vi "mainControlSerial.vi"(8 "error in (no error)":errorcluster, 10 "Queue In":T1) -> (0 "error out":errorcluster)   [LabVIEW 2014, in "LibraryGcode.lvlib"]
uses:
  LibraryGcode.lvlib
  control/Queue/QueueCMDandPOS.ctl
  control/Queue/TypeDataPOS.ctl
  control/stateCmdUpdatePara.ctl
  <vilib>/Platform/TimedLoop/XDataNode/timing_clust.ctl
  <vilib>/Platform/TimedLoop/XDataNode/nitl_modes.ctl
  <vilib>/Platform/TimedLoop/XDataNode/wakeup.ctl
  ClassUART/GiaoTiepUART.lvclass
  control/TypeFirmwareControl.ctl
  ClassUART/StateMachine_UART.ctl
  variableGlobal/StartAutoandGcode.vi
  <vilib>/Platform/TimedLoop/XDataNode/XDataNode.xnode
  <vilib>/Platform/TimedLoop/XDataNode/XDNodeRunTimeDep.lvlib
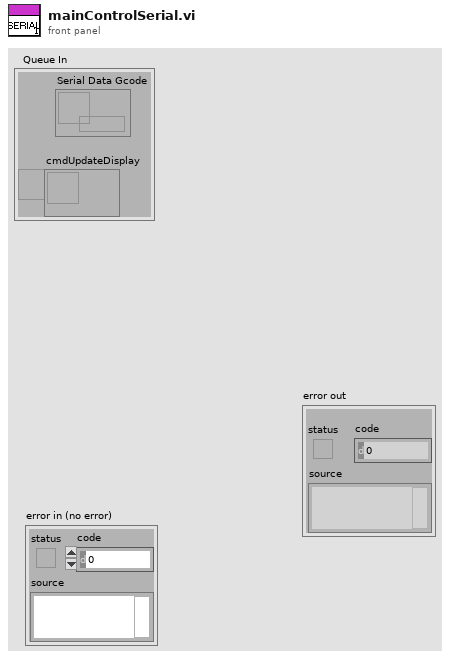
[diagram p1: front panel]
types:
  T1 = typedef "LibraryGcode.lvlib/QueueCMDandPOS.ctl" = cluster{"Serial Data Gcode":refnum<queue>, "cmdUpdateDisplay":refnum<queue>}
  T2 = typedef "LibraryGcode.lvlib/TypeFirmwareControl.ctl" = enum16{"ScaraMarlin", "CncMarlin", "Mk4Due"}
  T3 = typedef "XDNodeRunTimeDep.lvlib/timing_clust.ctl" = cluster{"Expected End [f-1]":u64, "Actual End [f-1]":u64, "Finished Late? [f-1]":bool, "Expected End [i-1]":u64, "Actual End [i-1]":u64, "Finished Late? [i-1]":bool, "Expected Start [i]":u64, "Actual Start [i]":u64, "Expected Start [f]":u64, "Actual Start [f]":u64, "Source Name":string, "Structure Name":string, "Period":i64, "Deadline":i64, "Offset":i64, "Start":i64, "Priority":i32, "Timeout":i32, "Mode":T4, "Wakeup Reason":T5, "Error":errorcluster, "Source Type":string, "Secondary Source Type":string, "Global End Time":u64, "Global Start Time":u64, "Frame Duration":u64, "Iteration Duration":u64, "Assigned CPU":i32, "I/O Scan Engine Mode":u32}
  T4 = typedef "XDNodeRunTimeDep.lvlib/nitl_modes.ctl" = enum32{"No Change", "Process missed periods, maintain original phase", "Discard missed periods, maintain original phase", "Process missed periods, ignore original phase", "Discard missed periods, ignore original phase"}
  T5 = typedef "XDNodeRunTimeDep.lvlib/wakeup.ctl" = enum32{"Normal", "Aborted", "Asynchronous wakeup", "Timing source error", "Timed loop error", "Timeout"}
  T6 = typedef "LibraryGcode.lvlib/GiaoTiepUART.lvclass/StateMachine_UART.ctl" = enum16{"INIT", "WRITE", "READ", "CHECKDATA", "IDLE", "STOP"}
  T7 = typedef "LibraryGcode.lvlib/stateBoardFirmware.ctl" = enum16{"Running", "Waiting", "Pos", "IDLE"}
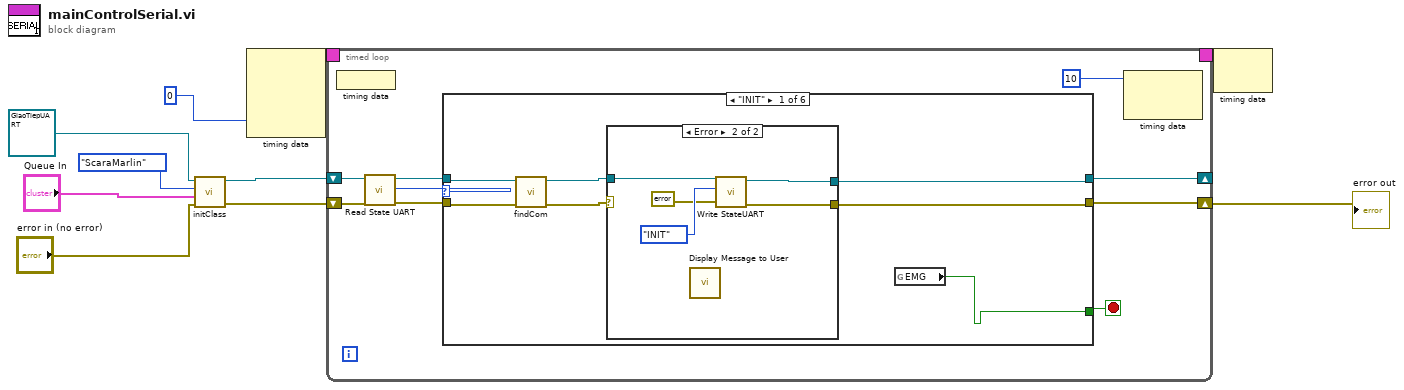
[diagram p0: block diagram]
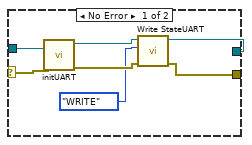
[diagram p2: hidden frame]
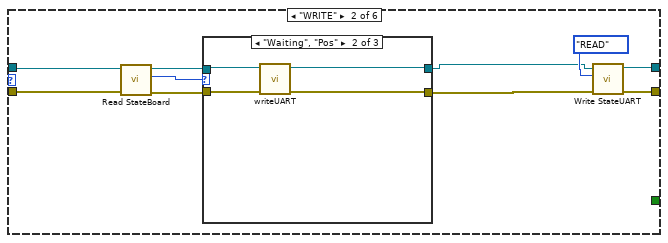
[diagram p3: hidden frame]
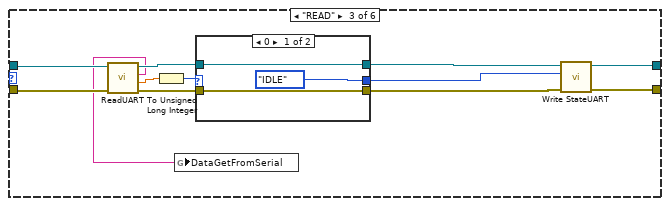
[diagram p6: hidden frame]
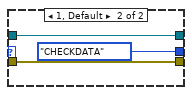
[diagram p7: hidden frame]
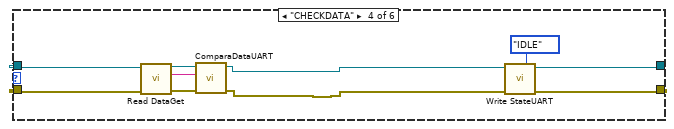
[diagram p8: hidden frame]
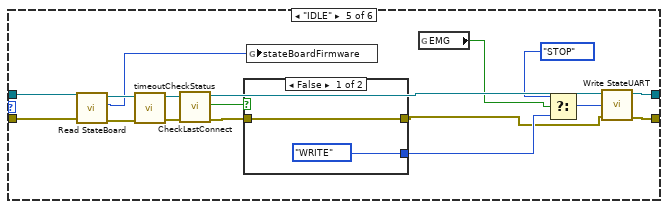
[diagram p9: hidden frame]
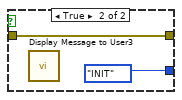
[diagram p10: hidden frame]
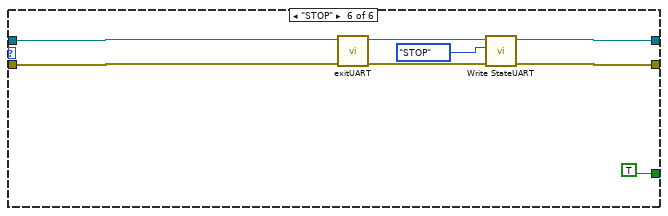
[diagram p11: hidden frame]
diagram:
  n1 = call-dynamic "initClass.vi"("error un"="error in (no error)", "Queue In"="Queue In", "TypeFirmware"=TypeFirmwareControl."ScaraMarlin", "GiaoTiepUART in"=refnum<class "GiaoTiepUART.lvclass"> refnum) -> ("error out"=w5:errorcluster, "GiaoTiepUART out"=w6:refnum<class "GiaoTiepUART.lvclass">)  [unwired: 6 in]
  n2 = node-c288(0 ("Processor")) -> (w10:T3)  [unwired: 3 in]
  n3 = timed-loop {
    timing: w10 -> [_]
    timing-out: [_] -> w9
    shift-right: [w18] -> _
    shift-left: w6 -> [w15]
    shift-right: [w17] -> w7
    shift-left: w5 -> [w16]
    stop <- w11 stop-if-true
    n4 = node-c288() -> ()  [unwired: 1 in]
    n5 = call-dynamic "Read State UART.vi"("error in (no error)"=w16, "GiaoTiepUART in"=w15) -> ("error out"=w13:errorcluster, "STATEUART"=w12:T6, "GiaoTiepUART out"=w14:refnum<class "GiaoTiepUART.lvclass">)  [unwired: 7 in]
    n6 = case shown="\"INIT\"" w12 {
      tunnel: [w20 _ _ _ _ TRUE] -> w11
      tunnel: [w26 w47 w66 w84 w97 w113] -> w18
      tunnel: w14 -> [w23 w42 w68 w81 w91 w106]
      tunnel: w13 -> [w22 w41 w67 w80 w89 w108]
      tunnel: [w21 w46 w65 w83 w96 w109] -> w17
      frame "INIT" {
        n7 = call-dynamic "findCom.vi"("error in (no error)"=w22, "GiaoTiep in"=w23) -> ("error out"=w25:errorcluster, "GiaoTiep out"=w24:refnum<class "GiaoTiepUART.lvclass">)  [unwired: 8 in]
        n8 = case shown="Error" w25 {
          selector: w25 -> [w33 _]
          tunnel: [w30 w36] -> w26
          tunnel: w24 -> [w32 w38]
          tunnel: [w31 w35] -> w21
          frame No Error {
            n9 = call-dynamic "initUART.vi"("error in (no error)"=w33, "GiaoTiep in"=w32) -> ("error out"=w28:errorcluster, "GiaoTiep out"=w29:refnum<class "GiaoTiepUART.lvclass">)  [unwired: 8 in]
            n10 = call-dynamic "Write StateUART.vi"("error in (no error)"=w28, "STATEUART"=StateMachine_UART."WRITE", "GiaoTiepUART in"=w29) -> ("error out"=w31:errorcluster, "GiaoTiepUART out"=w30:refnum<class "GiaoTiepUART.lvclass">)  [unwired: 7 in]
          }
          frame Error {
            n11 = call "Display Message to User"() -> ()  [unwired: 10 in, 2 out]
            n12 = call-dynamic "Write StateUART.vi"("error in (no error)"=errorcluster {"status"=FALSE, "code"=30011991, "source"="NoConnect "}, "STATEUART"=StateMachine_UART."INIT", "GiaoTiepUART in"=w38) -> ("error out"=w35:errorcluster, "GiaoTiepUART out"=w36:refnum<class "GiaoTiepUART.lvclass">)  [unwired: 7 in]
          }
        }
        n13 = global read "StartAutoandGcode.vi" "EMG"() -> (w20:bool)
      }
      frame "WRITE" {
        n14 = call-dynamic "Read StateBoard.vi"("error in (no error)"=w41, "XuLyStringUART in"=w42) -> ("error out"=w43:errorcluster, "StatePos"=w40:T7, "XuLyStringUART out"=w44:refnum<class "GiaoTiepUART.lvclass">)  [unwired: 7 in]
        n15 = case shown="\"Waiting\", \"Pos\"" w40 {
          tunnel: w44 -> [w50 w54 w56]
          tunnel: [w50 w52 w56] -> w39
          tunnel: w43 -> [w49 w53 w55]
          tunnel: [w49 w51 w55] -> w48
          frame "Running", Default {
          }
          frame "Waiting", "Pos" {
            n16 = call-dynamic "writeUART.vi"("error in (no error)"=w53, "GiaoTiep in"=w54) -> ("error out"=w51:errorcluster, "GiaoTiep out"=w52:refnum<class "GiaoTiepUART.lvclass">)  [unwired: 7 in, 1 out]
          }
          frame "IDLE" {
          }
        }
        n17 = call-dynamic "Write StateUART.vi"("error in (no error)"=w48, "STATEUART"=StateMachine_UART."READ", "GiaoTiepUART in"=w39) -> ("error out"=w46:errorcluster, "GiaoTiepUART out"=w47:refnum<class "GiaoTiepUART.lvclass">)  [unwired: 7 in]
      }
      frame "READ" {
        n18 = call-dynamic "ReadUART.vi"("error in (no error)"=w67, "GiaoTiep in"=w68) -> ("error out"=w62:errorcluster, "milisecondGetData"=w59:dbl, "read buffer"=w57:string, "GiaoTiep out"=w61:refnum<class "GiaoTiepUART.lvclass">)  [unwired: 6 in]
        n19 = To Unsigned Long Integer(number=w59) -> (unsigned 32bit integer=w58:u32)
        n20 = global write "StartAutoandGcode.vi" "DataGetFromSerial"(w57) -> ()
        n21 = case shown="0" w58 {
          tunnel: [StateMachine_UART."IDLE" StateMachine_UART."CHECKDATA"] -> w64
          tunnel: [w70 w73] -> w63
          tunnel: w62 -> [w70 w73]
          tunnel: [w69 w72] -> w60
          tunnel: w61 -> [w69 w72]
          frame 0 {
          }
          frame 1, Default {
          }
        }
        n22 = call-dynamic "Write StateUART.vi"("error in (no error)"=w63, "STATEUART"=w64, "GiaoTiepUART in"=w60) -> ("error out"=w65:errorcluster, "GiaoTiepUART out"=w66:refnum<class "GiaoTiepUART.lvclass">)  [unwired: 7 in]
      }
      frame "CHECKDATA" {
        n23 = call-dynamic "Read DataGet.vi"("error in (no error)"=w80, "GiaoTiepUART in"=w81) -> ("error out"=w78:errorcluster, "DataGet"=w77:string, "GiaoTiepUART out"=w79:refnum<class "GiaoTiepUART.lvclass">)  [unwired: 7 in]
        n24 = call-dynamic "ComparaDataUART.vi"("error in (no error)"=w78, "StringIN"=w77, "XuLyStringUART in"=w79) -> ("error out"=w75:errorcluster, "XuLyStringUART out"=w76:refnum<class "GiaoTiepUART.lvclass">)  [unwired: 7 in]
        n25 = call-dynamic "Write StateUART.vi"("error in (no error)"=w75, "STATEUART"=StateMachine_UART."IDLE", "GiaoTiepUART in"=w76) -> ("error out"=w83:errorcluster, "GiaoTiepUART out"=w84:refnum<class "GiaoTiepUART.lvclass">)  [unwired: 7 in]
      }
      frame "IDLE" {
        n26 = call-dynamic "Read StateBoard.vi"("error in (no error)"=w89, "XuLyStringUART in"=w91) -> ("error out"=w88:errorcluster, "StatePos"=w87:T7, "XuLyStringUART out"=w90:refnum<class "GiaoTiepUART.lvclass">)  [unwired: 7 in]
        n27 = call-dynamic "timeoutCheckStatus.vi"("error in (no error)"=w88, "GiaoTiepUART in"=w90) -> ("error out"=w98:errorcluster, "GiaoTiepUART out"=w101:refnum<class "GiaoTiepUART.lvclass">)  [unwired: 8 in]
        n28 = call-dynamic "CheckLastConnect.vi"("error in (no error)"=w98, "GiaoTiepUART in"=w101) -> ("error out"=w92:errorcluster, "timeOut"=w100:bool, "GiaoTiepUART out"=w95:refnum<class "GiaoTiepUART.lvclass">)  [unwired: 7 in]
        n29 = case shown="False" w100 {
          tunnel: [StateMachine_UART."WRITE" StateMachine_UART."INIT"] -> w99
          tunnel: [w102 w104] -> w86
          tunnel: w92 -> [w102 w104]
          frame False {
          }
          frame True {
            n30 = call "Display Message to User3"() -> ()  [unwired: 10 in, 2 out]
          }
        }
        n31 = global write "StartAutoandGcode.vi" "stateBoardFirmware"(w87) -> ()
        n32 = global read "StartAutoandGcode.vi" "EMG"() -> (w85:bool)
        n33 = Select(t=StateMachine_UART."STOP", s=w85, f=w99) -> (s? t:f=w94:T6)
        n34 = call-dynamic "Write StateUART.vi"("error in (no error)"=w86, "STATEUART"=w94, "GiaoTiepUART in"=w95) -> ("error out"=w96:errorcluster, "GiaoTiepUART out"=w97:refnum<class "GiaoTiepUART.lvclass">)  [unwired: 7 in]
      }
      frame "STOP" {
        (unwired) TRUE
        n35 = call-dynamic "exitUART.vi"("error in (no error)"=w108, "GiaoTiep in"=w106) -> ("error out"=w110:errorcluster, "GiaoTiep out"=w111:refnum<class "GiaoTiepUART.lvclass">)  [unwired: 8 in]
        n36 = call-dynamic "Write StateUART.vi"("error in (no error)"=w110, "STATEUART"=StateMachine_UART."STOP", "GiaoTiepUART in"=w111) -> ("error out"=w109:errorcluster, "GiaoTiepUART out"=w113:refnum<class "GiaoTiepUART.lvclass">)  [unwired: 7 in]
      }
    }
    n37 = node-c288(i64 10 ("Period")) -> ()  [unwired: 1 in, 1 out]
  }
  "error out" <- w7
  n38 = node-c288(w9) -> ()  [unwired: 1 out]
